vi "QUDI_QPD_PID_laser_control.vi"() -> ()   [LabVIEW 2015]
uses:
  <vilib>/rvi/Analysis/control/PID/Typedef/niFpgaPID_PIGains.ctl
  <vilib>/Platform/TimedLoop/XDataNode/timing_clust.ctl
  <vilib>/Platform/TimedLoop/XDataNode/nitl_modes.ctl
  <vilib>/Platform/TimedLoop/XDataNode/wakeup.ctl
  <vilib>/rvi/FXPMathLib/basic elements/FxpIntAccumulator/subVIs/nifxpmath_IntAccumulator_SimConfig.ctl
  <vilib>/rvi/Emulation/niFpgaGetClockAttributes.vi
  <vilib>/rvi/Emulation/niFpgaSctlEmulationGetInTimedLoop.vi
  <vilib>/rvi/Emulation/niFpgaEmulationReportErrorSimple.vi
  <vilib>/rvi/Emulation/niFpgaProcessEmulError.vi
  <vilib>/rvi/eio/common/nirviEmuTemplateMethod_errors.vi
  <vilib>/rvi/Analysis/common/codeGenErrors/XNode/niFpgaXNodeCodeGenErrorHandle.vi
  <vilib>/rvi/Emulation/niFpgaCriticalErrorInLSC.vi
  <vilib>/rvi/FXPMathLib/basic elements/FxpIntAccumulator/simVIs/DllFxpIntAccumulator_sub.vi
  <vilib>/rvi/Analysis/control/PID/SubVIs/niFpgaPID_PIWrapper.vi
  <vilib>/eio/EIONode/EIONode.xnode
  <vilib>/rvi/Analysis/measure/dc-rms/XNode/niFpgaDC-RMS.xnode
  <vilib>/Platform/TimedLoop/XDataNode/XDataNode.xnode
  <vilib>/rvi/FXPMathLib/basic elements/FxpIntAccumulator/XNode/nifxpmath_IntAccumulator.xnode
  <vilib>/Platform/TimedLoop/XDataNode/XDNodeRunTimeDep.lvlib
panel:
  in  "ref_axis":bool
  out "output":i16
  in  "I":i16
  in  "P":i16
  in  "reset":bool
  in  "setpoint":i16
  in  "autofocus":bool
  out "counter":u32
  out "Sum":i16
  out "Y":i16
  out "X":i16
  in  "561":i16
  in  "640":i16
  in  "405":i16
  in  "488":i16
  in  "integration_time_us":u32=100 caption="Count(uSec)"
  in  "stop":bool
  out "duration_ms":u32
  in  "reset_counter":bool
  in  "Update lasers":bool
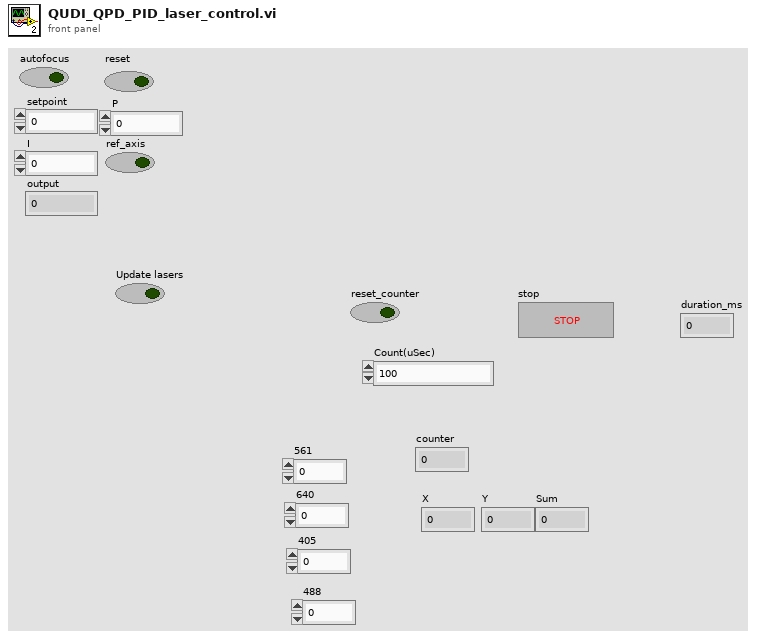
[diagram p1: front panel]
types:
  T1 = typedef "niFpgaPID_PIGains.ctl" = cluster{"proportional gain":sgl, "integral gain":sgl}
  T2 = typedef "XDNodeRunTimeDep.lvlib/timing_clust.ctl" = cluster{"Expected End [f-1]":u64, "Actual End [f-1]":u64, "Finished Late? [f-1]":bool, "Expected End [i-1]":u64, "Actual End [i-1]":u64, "Finished Late? [i-1]":bool, "Expected Start [i]":u64, "Actual Start [i]":u64, "Expected Start [f]":u64, "Actual Start [f]":u64, "Source Name":string, "Structure Name":string, "Period":i64, "Deadline":i64, "Offset":i64, "Start":i64, "Priority":i32, "Timeout":i32, "Mode":T3, "Wakeup Reason":T4, "Error":errorcluster, "Source Type":string, "Secondary Source Type":string, "Global End Time":u64, "Global Start Time":u64, "Frame Duration":u64, "Iteration Duration":u64, "Assigned CPU":i32, "I/O Scan Engine Mode":u32}
  T3 = typedef "XDNodeRunTimeDep.lvlib/nitl_modes.ctl" = enum32{"No Change", "Process missed periods, maintain original phase", "Discard missed periods, maintain original phase", "Process missed periods, ignore original phase", "Discard missed periods, ignore original phase"}
  T4 = typedef "XDNodeRunTimeDep.lvlib/wakeup.ctl" = enum32{"Normal", "Aborted", "Asynchronous wakeup", "Timing source error", "Timed loop error", "Timeout"}
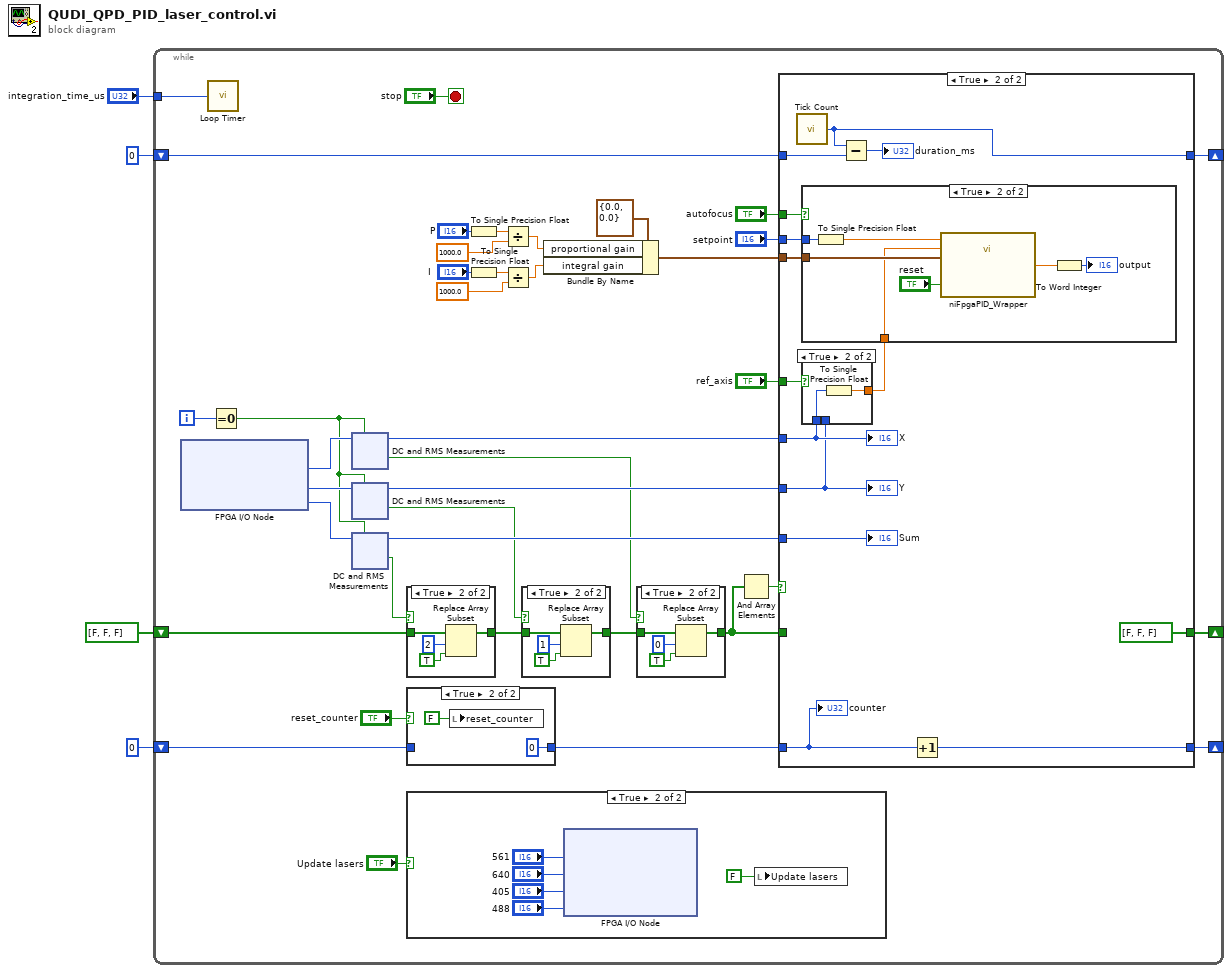
[diagram p0: block diagram]
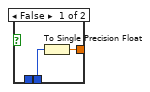
[diagram p8: hidden frame]
diagram:
  n1 = while {
    shift-right: [w26] -> _
    shift-left: bool[] [FALSE, FALSE, FALSE] ("initialized array") -> [w34]
    shift-right: [w24] -> _
    shift-left: u32 0 -> [w25]
    tunnel: "integration_time_us" -> [w23]
    shift-right: [w22] -> _
    shift-left: u32 0 -> [w20]
    i -> [w41]
    stop <- "stop" stop-if-true
    n2 = xnode "FPGA I/O Node"() -> ("Connector0/AI0"=w43:i16, "Connector0/AI1"=w39:i16, "Connector0/AI2"=w38:i16)  [unwired: 3 in, 3 out]
    n3 = call "Loop Timer"("Count(uSec)"=w23) -> ()  [unwired: 1 out]
    n4 = Equal To 0?(x=w41) -> (x = 0?=w35:bool)
    n5 = xnode "DC and RMS Measurements"("input data"=w43, "reset"=w35) -> ("DC"=w40:i16, "output valid"=w29:bool)
    n6 = xnode "DC and RMS Measurements"("input data"=w39, "reset"=w35) -> ("DC"=w37:i16, "output valid"=w30:bool)
    n7 = xnode "DC and RMS Measurements"("input data"=w38, "reset"=w35) -> ("DC"=w36:i16, "output valid"=w31:bool)
    n8 = case shown="True" w31 {
      tunnel: w34 -> [w57 w60]
      tunnel: [w57 w58] -> w33
      frame False {
      }
      frame True {
        n9 = Replace Array Subset(array=w60, new element=TRUE, index=2) -> (w58:bool[])
      }
    }
    n10 = case shown="True" "reset_counter" {
      tunnel: w20 -> [w49 _]
      tunnel: [w49 u32 0] -> w19
      frame False {
      }
      frame True {
        n11 = local write "reset_counter"(FALSE ("Reset counter")) -> ()
      }
    }
    n12 = case shown="True" "Update lasers" {
      frame False {
      }
      frame True {
        n13 = xnode "FPGA I/O Node"("Connector0/AO0"="561", "Connector0/AO1"="640", "Connector0/AO2"="405", "Connector0/AO3"="488") -> ()  [unwired: 4 in, 4 out]
        n14 = local write "Update lasers"(FALSE ("Update lasers")) -> ()
      }
    }
    n15 = To Single Precision Float(number="P") -> (single precision float=w11:sgl)
    n16 = To Single Precision Float(number="I") -> (single precision float=w8:sgl)
    n17 = Divide(x=w11, y=sgl 1000.0) -> (x/y=w9:sgl)
    n18 = Divide(x=w8, y=sgl 1000.0) -> (x/y=w6:sgl)
    n19 = case shown="True" w30 {
      tunnel: w33 -> [w62 w65]
      tunnel: [w62 w63] -> w32
      frame False {
      }
      frame True {
        n20 = Replace Array Subset(array=w65, new element=TRUE, index=1) -> (w63:bool[])
      }
    }
    n21 = Bundle By Name(cluster=T1 {"proportional gain"=0.0, "integral gain"=0.0} ("gains"), "proportional gain"=w9, "integral gain"=w6) -> (w12:T1)
    n22 = case shown="True" w29 {
      tunnel: [w52 w54] -> w27
      tunnel: w32 -> [w52 w53]
      frame False {
      }
      frame True {
        n23 = Replace Array Subset(array=w53, new element=TRUE, index=0) -> (w54:bool[])
      }
    }
    n24 = And Array Elements(Boolean array=w27) -> (logical AND=w28:bool)
    n25 = case shown="True" w28 {
      tunnel: w40 -> [_ w72]
      tunnel: w37 -> [_ w70]
      tunnel: w36 -> [_ w78]
      tunnel: w27 -> [w69 _]
      tunnel: [w69 bool[] [FALSE, FALSE, FALSE] ("initialized array")] -> w26
      tunnel: w25 -> [w68 w82]
      tunnel: [w68 w80] -> w24
      tunnel: w19 -> [w67 w77]
      tunnel: [w67 w79] -> w22
      tunnel: "autofocus" -> [_ w76]
      tunnel: "setpoint" -> [_ w75]
      tunnel: w12 -> [_ w74]
      tunnel: "ref_axis" -> [_ w73]
      frame False {
      }
      frame True {
        n26 = call "Tick Count"() -> ("Tick Count(mSec)"=w80:u32)
        n27 = case shown="True" w73 {
          tunnel: w72 -> [_ w87]
          tunnel: [w84 w86] -> w71
          tunnel: w70 -> [w85 _]
          frame False {
            n28 = To Single Precision Float(number=w85) -> (single precision float=w84:sgl)
          }
          frame True {
            n29 = To Single Precision Float(number=w87) -> (single precision float=w86:sgl)
          }
        }
        n30 = case shown="True" w76 {
          tunnel: w75 -> [_ w94]
          tunnel: w74 -> [_ w92]
          tunnel: w71 -> [_ w88]
          frame False {
          }
          frame True {
            n31 = To Single Precision Float(number=w94) -> (single precision float=w93:sgl)
            n32 = call-poly <vilib>:"niFpgaPID_Wrapper.vi"("setpoint"=w93, "reset? (F)"="reset", "process variable"=w88, "gains"=w92) -> ("output"=w90:sgl)  [unwired: 9 in, 2 out]
            n33 = To Word Integer(number=w90) -> (16bit integer=→"output":i16)
          }
        }
        n34 = Subtract(x=w80, y=w82) -> (x-y=→"duration_ms":u32)
        n35 = Increment(x=w77) -> (x+1=w79:u32)
        "X" <- w72
        "Y" <- w70
        "Sum" <- w78
        "counter" <- w77
      }
    }
  }
